vi "OE1022DRandXita.vi"(2 "Y":dbl, 3 "X":dbl) -> (0 "θ (°)":dbl, 1 "R":dbl)   [LabVIEW 2022 SP3]
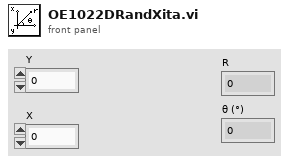
[diagram p1: front panel]
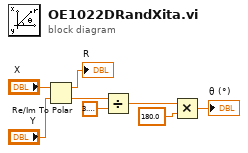
[diagram p0: block diagram]
diagram:
  n1 = Re/Im To Polar(2:"Y", 3:"X") -> (0:w2:dbl, 1:→"R":dbl)
  n2 = Divide(x=w2, y=3.141592653589793) -> (x/y=w7:dbl)
  n3 = Multiply(x=w7, y=180.0) -> (x*y=→"θ (°)":dbl)
